vi "CreateEvents.vi"(8 "error in (no error)":errorcluster, 11 "NewTemplate in":refnum<class "UIManager.lvclass">) -> (0 "error out":errorcluster, 3 "NewTemplate out":refnum<class "UIManager.lvclass">)   [LabVIEW 2024, in "UIManager.lvclass"]
uses:
  UIManager.lvclass
  UIManager.lvclass/UIManager.ctl
  JQMHCore/Module/RQMHModule.lvclass
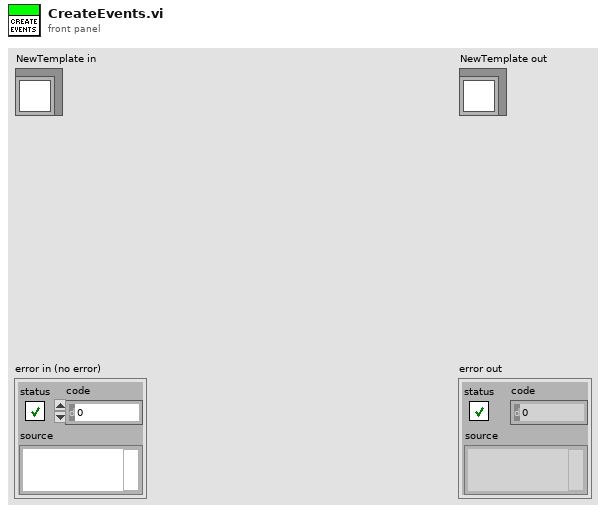
[diagram p1: front panel]
types:
  T1 = typedef "UIManager.lvclass/Broadcast Events--cluster.ctl" = cluster{"Stopped":refnum<user-event>, "Request Stop":refnum<user-event>}
  T2 = typedef "UIManager.lvclass/Request Events--cluster.ctl" = cluster{"Do Something":refnum<user-event>}
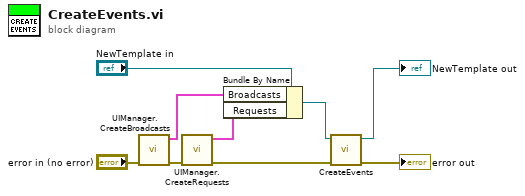
[diagram p0: block diagram]
diagram:
  n1 = call "UIManager.CreateBroadcasts.vi"("error in (no error)"="error in (no error)") -> ("error out"=w3:errorcluster, "Broadcasts"=w1:T1)  [unwired: 9 in]
  n2 = call "UIManager.CreateRequests.vi"("error in (no error)"=w3) -> ("error out"=w2:errorcluster, "Requests"=w4:T2)  [unwired: 9 in]
  n3 = Bundle By Name(cluster="NewTemplate in", "Broadcasts"=w1, "Requests"=w4) -> (w6:refnum<class "UIManager.lvclass">)
  n4 = call-parent "CreateEvents.vi"("error in (no error)"=w2, "JQMHCore in"=w6) -> ("error out"=→"error out":errorcluster, "JQMHCore out"=→"NewTemplate out":refnum<class "UIManager.lvclass">)  [unwired: 8 in]
